vi "Main_Module.vi"(11 "Error_In":errorcluster) -> (15 "Error_Out":errorcluster)   [LabVIEW 2021]
doc: "This is the Main VI for the user to interact with."
uses:
  Controls/Queue_Operation.ctl
  Controls/Logger_Data.ctl
  Controls/Temperature_Limit.ctl
  Controls/Current_Limit.ctl
  Controls/Generated_data.ctl
  Controls/Main_Status.ctl
panel:
  in  "Log_Rate":dbl=1.0 min=1.0 max=120.0
  out "Temperature":dbl
  out "Current":dbl
  out "Generated_Data":dbl[][](graph)
  in  "Exit":bool
  in  "Current_Limit":T1={"Current_High_Limit"=120.0, "Current_Low_Limit"=0.0} caption="Current Limit" {"Current_High_Limit" min=101.0 max=120.0; "Current_Low_Limit" min=100.0 max=119.0}
  in  "Temperature_Limit":T2={"Temperature_High_Limit"=49.0, "Temperature_Low_Limit"=30.0} caption="Temperature Limit" {"Temperature_Low_Limit" min=30.0 max=49.0; "Temperature_High_Limit" min=31.0 max=50.0}
  in  "Start/Stop_Acquisition":bool caption="Start/Stop Acquisition"
  # "ADQ System"
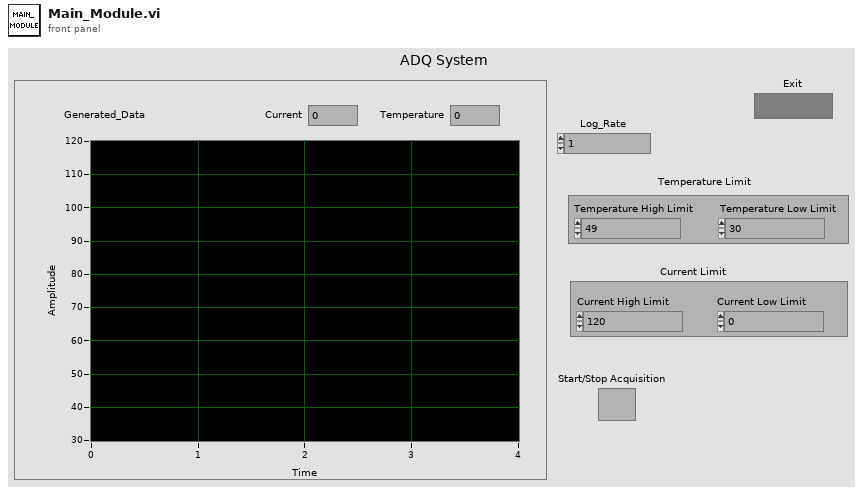
[diagram p1: front panel]
types:
  T1 = typedef "Current_Limit.ctl" = cluster{"Current_High_Limit":dbl, "Current_Low_Limit":dbl}
  T2 = typedef "Temperature_Limit.ctl" = cluster{"Temperature_High_Limit":dbl, "Temperature_Low_Limit":dbl}
  T3 = typedef "Main_Status.ctl" = cluster{"Stop?":bool, "Start/Stop_Acquisition ":bool, "Wait_Time":i32}
  T4 = typedef "Queue_Operation.ctl" = enum16{"Obtain_Queue", "Enqueue", "Lossy_Enqueue", "Preview", "Queue_Status", "Release_Queue", "Dequeue", "Flush"}
  T5 = enum8{"Enabled", "Disabled", "Disabled and Grayed Out"}
  T6 = typedef "Logger_Data.ctl" = cluster{"Generated_Data":T7, "Current_Limit":T1, "Temperature_Limit":T2}
  T7 = typedef "Generated_data.ctl" = cluster{"Current_Data":dbl, "Temp_Data":dbl}
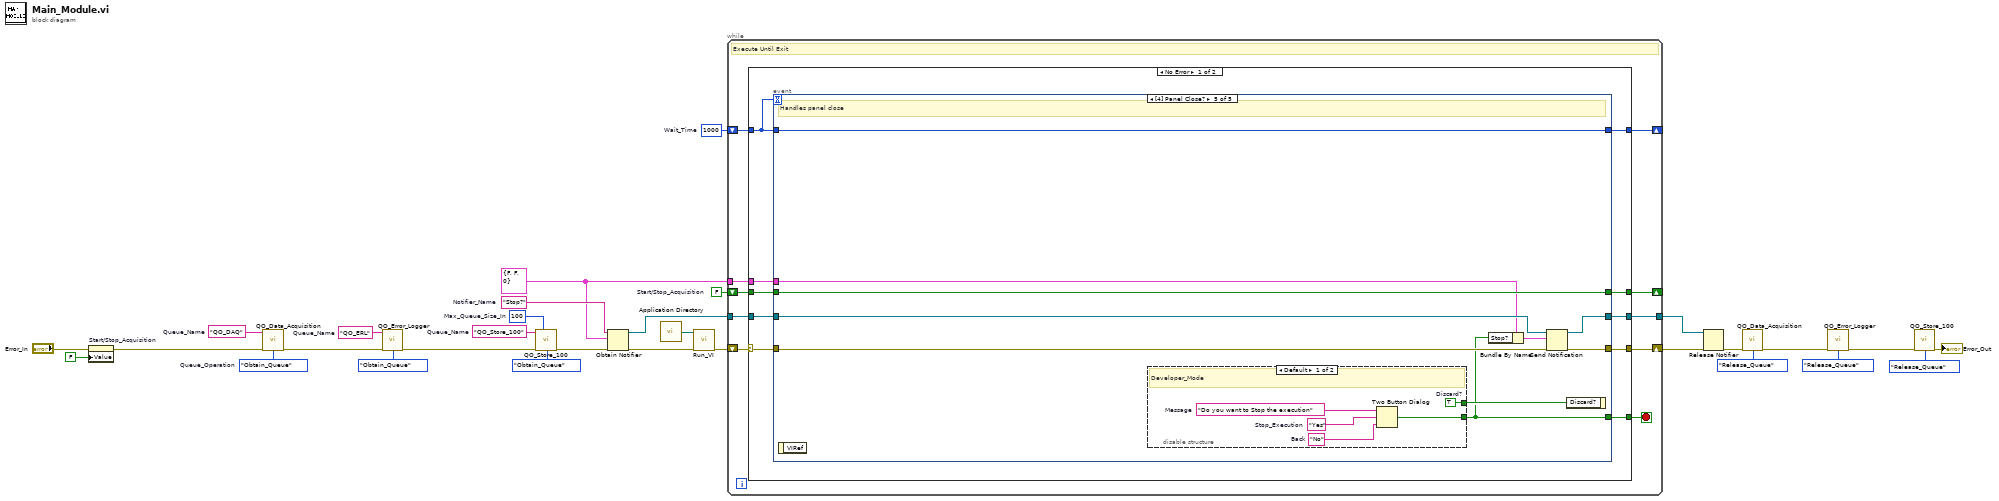
[diagram p0: block diagram]
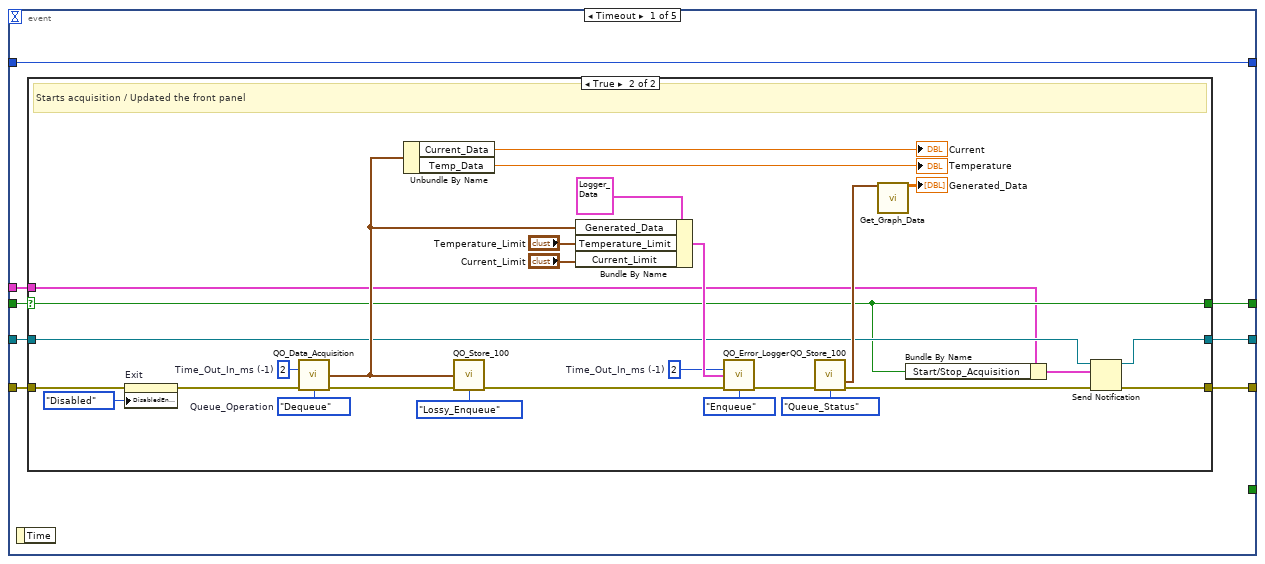
[diagram p2: hidden frame]
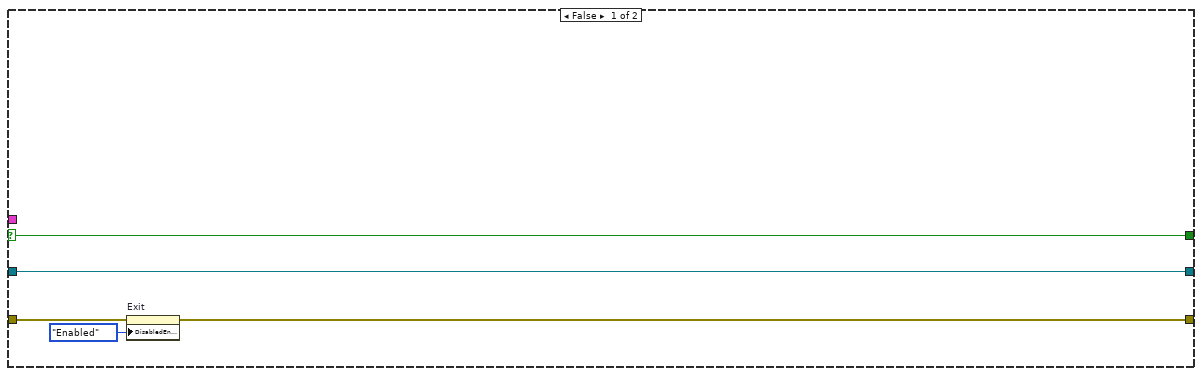
[diagram p3: hidden frame]
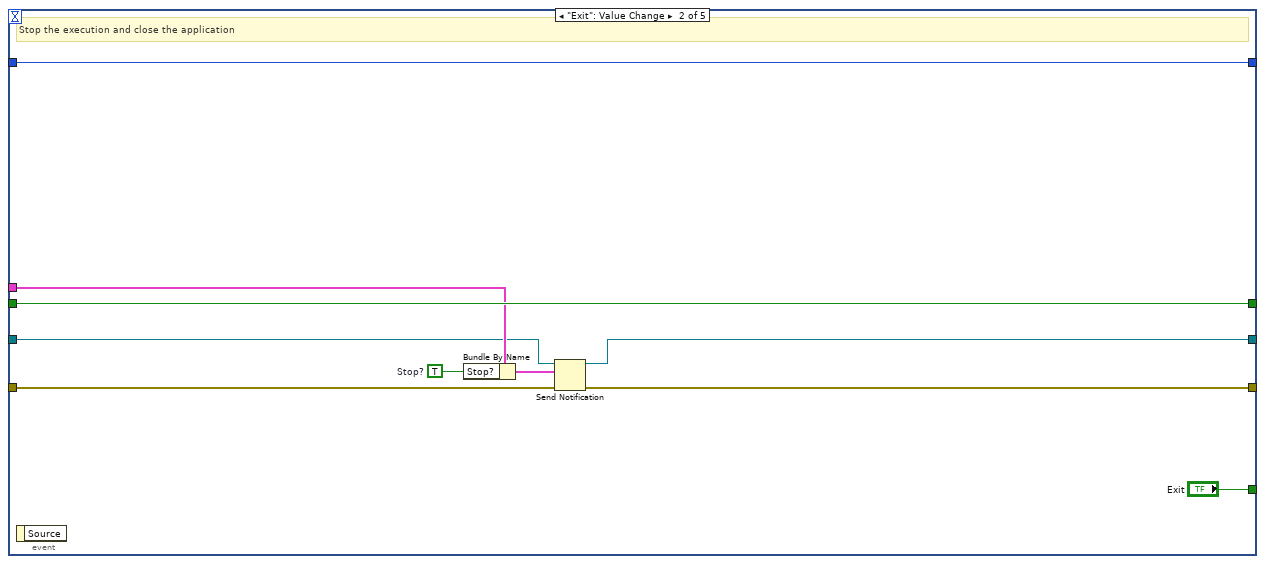
[diagram p4: hidden frame]
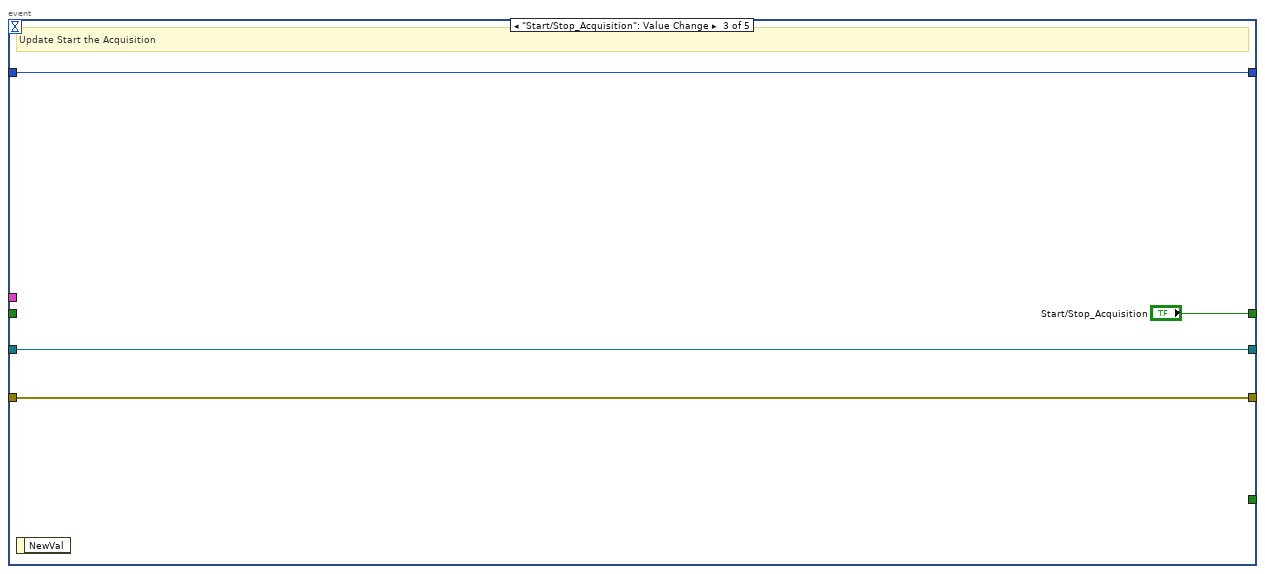
[diagram p5: hidden frame]
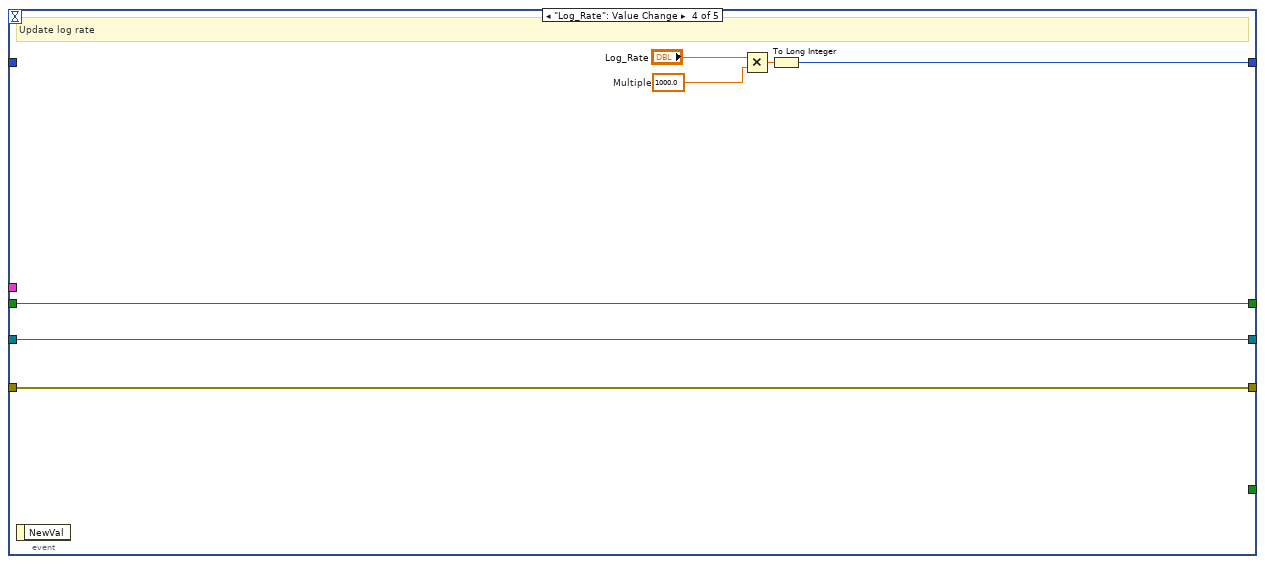
[diagram p6: hidden frame]
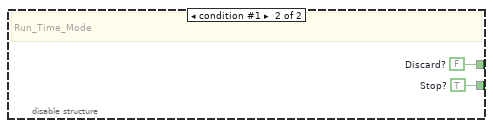
[diagram p7: hidden frame]
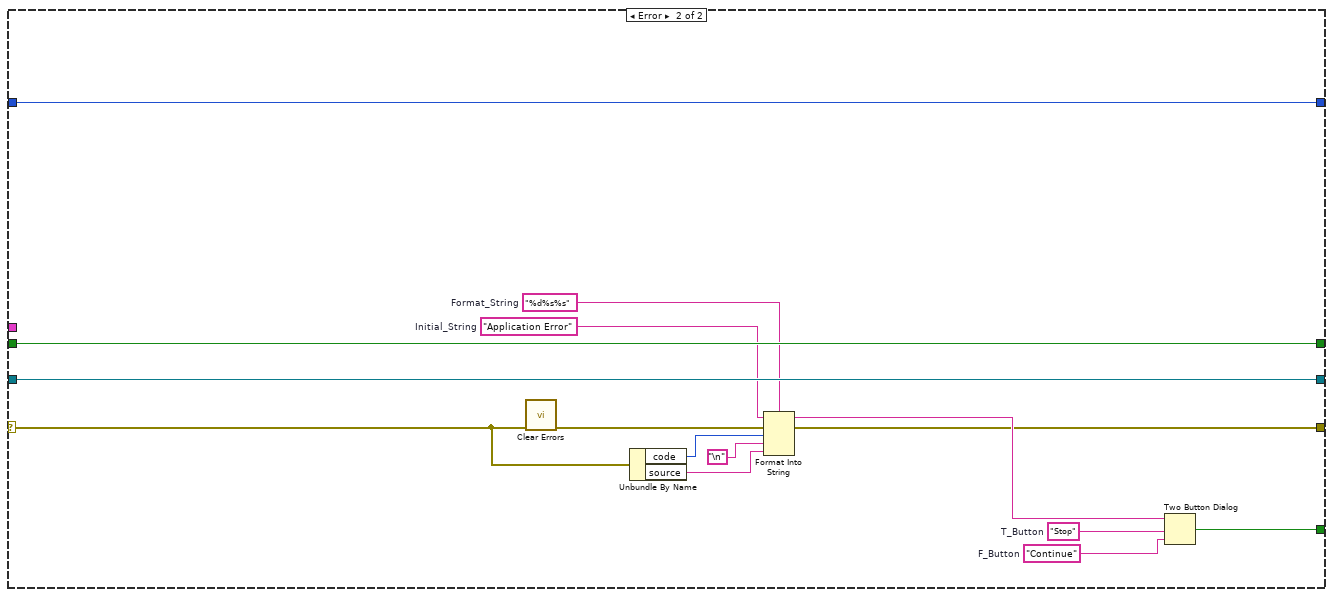
[diagram p8: hidden frame]
diagram:
  w2 = T3 {"Stop?"=FALSE, "Start/Stop_Acquisition "=FALSE, "Wait_Time"=0}
  w11 = "QO_Store_100"  # Queue_Name
  w12 = "QO_ERL"  # Queue_Name
  w13 = "QO_DAQ"  # Queue_Name
  w21 = "Stop?"  # Notifier_Name
  w27 = 1000  # Wait_Time
  w23 = 100  # Max_Queue_Size_In
  w28 = FALSE  # Start/Stop_Acquisition
  w29 = Queue_Operation."Obtain_Queue"  # Queue_Operation
  n1 = property on="Start/Stop_Acquisition" class="Bool (strict)"(error in="Error_In", "Value"=FALSE ("Start/Stop_Acquisition")) -> (error out=w10:errorcluster)  [unwired: 1 in, 1 out]
  n2 = call "QO_Data_Acquisition.vi"("Queue_Name_In"=w13, "Error_In"=w10, "Queue_Operation"=w29) -> ("Error_Out"=w30:errorcluster)  [unwired: 8 in, 4 out]
  n3 = call "QO_Error_Logger.vi"("Queue_Name_In"=w12, "Error_In"=w30, "Queue_Operation"=Queue_Operation."Obtain_Queue") -> ("Error_Out"=w26:errorcluster)  [unwired: 8 in, 4 out]
  n4 = call "QO_Store_100.vi"("Queue_Name_In"=w11, "Max_Queue_Size_In"=w23, "Error_In"=w26, "Queue_Operation"=Queue_Operation."Obtain_Queue") -> ("Error_Out"=w24:errorcluster)  [unwired: 7 in, 4 out]
  n5 = Obtain Notifier(name (unnamed)=w21, notification data type=w2, error in (no error)=w24) -> (notifier out=w20:refnum<notifier>, error out=w17:errorcluster)  [unwired: 1 in, 1 out]
  n6 = call <vilib>:"Application Directory.vi"() -> ("Application Directory"=w15:path)
  n7 = call "Run_VI.vi"("Application_Directory"=w15, "Error_In"=w17) -> ("Error_Out"=w16:errorcluster)  [unwired: 13 in]
  n8 = while {
    shift-right: [w38] -> _
    shift-left: w28 -> [w37]
    shift-right: [w35] -> _
    shift-left: w27 -> [w36]
    tunnel: w20 -> [w34]
    tunnel: [w33] -> w19
    tunnel: w2 -> [w32]
    shift-right: [w31] -> w1
    shift-left: w16 -> [w40]
    stop <- w39 stop-if-true
    # "Execute Until Exit"
    n9 = case shown="No Error" w40 {
      selector: w40 -> [w41 w131]
      tunnel: [w50 w130] -> w39
      tunnel: [w49 w144] -> w38
      tunnel: w37 -> [w48 w144]
      tunnel: [w47 w132] -> w31
      tunnel: w36 -> [w43 w143]
      tunnel: [w46 w143] -> w35
      tunnel: w34 -> [w42 w142]
      tunnel: [w44 w142] -> w33
      tunnel: w32 -> [w45 _]
      frame No Error {
        n10 = event shown="[4] Panel Close?" {
          selector: _ -> [_ _ _ _ _]
          dyn-events: _ -> [_ _ _ _ _]
          timeout: w43 -> [_ _ _ _ _]
          tunnel: [_ "Exit" _ _ w114] -> w50
          tunnel: [w57 w100 "Start/Stop_Acquisition" w106 w121] -> w49
          tunnel: w48 -> [w56 w100 _ w106 w121]
          tunnel: w41 -> [w54 w99 w105 w108 w120]
          tunnel: [w58 w97 w105 w108 w118] -> w47
          tunnel: [w55 w98 w104 w109 w119] -> w46
          tunnel: w43 -> [w55 w98 w104 _ w119]
          tunnel: w45 -> [w51 w94 _ _ w115]
          tunnel: w42 -> [w53 w93 w102 w107 w117]
          tunnel: [w52 w92 w102 w107 w113] -> w44
          event Timeout {
            n11 = event-data() -> ()  [unwired: 1 in, 1 out]
            n12 = case shown="True" w56 {
              selector: w56 -> [w62 w69]
              tunnel: w54 -> [w63 w91]
              tunnel: [w60 w73] -> w58
              tunnel: [w62 w69] -> w57
              tunnel: w53 -> [w61 w72]
              tunnel: [w61 w71] -> w52
              tunnel: w51 -> [_ w68]
              frame False {
                n13 = property on="Exit" class="Bool"(error in=w63, "DisabledEnum"=T5."Enabled" ("Disabled")) -> (error out=w60:errorcluster)  [unwired: 1 in, 1 out]
              }
              frame True {
                w75 = 2  # Time_Out_In_ms (-1)
                w76 = 2  # Time_Out_In_ms (-1)
                w90 = Queue_Operation."Dequeue"  # Queue_Operation
                # "Starts acquisition / Updated the front panel"
                n14 = property on="Exit" class="Bool"(error in=w91, "DisabledEnum"=T5."Disabled" ("Disabled")) -> (error out=w65:errorcluster)  [unwired: 1 in, 1 out]
                n15 = call "QO_Data_Acquisition.vi"("Time_Out_In_ms (-1)"=w76, "Error_In"=w65, "Queue_Operation"=w90) -> ("Data_Out"=w80:T7, "Error_Out"=w88:errorcluster)  [unwired: 8 in, 3 out]
                n16 = Unbundle By Name(w80) -> ("Current_Data"=→"Current":dbl, "Temp_Data"=→"Temperature":dbl)
                n17 = call "QO_Store_100.vi"("Data_In"=w80, "Error_In"=w88, "Queue_Operation"=Queue_Operation."Lossy_Enqueue") -> ("Error_Out"=w77:errorcluster)  [unwired: 8 in, 4 out]
                n18 = Bundle By Name(cluster=T6 {"Generated_Data"={"Current_Data"=0.0, "Temp_Data"=0.0}, "Current_Limit"={"Current_High_Limit"=0.0, "Current_Low_Limit"=0.0}, "Temperature_Limit"={"Temperature_High_Limit"=0.0, "Temperature_Low_Limit"=0.0}} ("Logger_Data"), "Generated_Data"=w80, "Temperature_Limit"="Temperature_Limit", "Current_Limit"="Current_Limit") -> (w82:T6)
                n19 = call "QO_Error_Logger.vi"("Time_Out_In_ms (-1)"=w75, "Data_In"=w82, "Error_In"=w77, "Queue_Operation"=Queue_Operation."Enqueue") -> ("Error_Out"=w84:errorcluster)  [unwired: 7 in, 4 out]
                n20 = call "QO_Store_100.vi"("Error_In"=w84, "Queue_Operation"=Queue_Operation."Queue_Status") -> ("Total_Data"=w85:T7[], "Error_Out"=w74:errorcluster)  [unwired: 9 in, 3 out]
                n21 = call "Get_Graph_Data.vi"("Total_Data"=w85) -> ("Array"=→"Generated_Data":dbl[][])  [unwired: 14 in]
                n22 = Bundle By Name(cluster=w68, "Start/Stop_Acquisition"=w69) -> (w70:T3)
                n23 = Send Notification(notification=w70, notifier=w72, error in (no error)=w74) -> (notifier out=w71:refnum<notifier>, error out=w73:errorcluster)
              }
            }
          }
          event "Exit": Value Change {
            w96 = TRUE  # Stop?
            # "Stop the execution and close the application"
            n24 = event-data() -> ()  [unwired: 1 in, 1 out]
            n25 = Bundle By Name(cluster=w94, "Stop?"=w96) -> (w95:T3)
            n26 = Send Notification(notification=w95, notifier=w93, error in (no error)=w99) -> (notifier out=w92:refnum<notifier>, error out=w97:errorcluster)
          }
          event "Start/Stop_Acquisition": Value Change {
            # "Update Start the Acquisition"
            n27 = event-data() -> ()  [unwired: 1 in, 1 out]
          }
          event "Log_Rate": Value Change {
            w111 = 1000.0  # Multiple
            # "Update log rate"
            n28 = event-data() -> ()  [unwired: 1 in, 1 out]
            n29 = Multiply(x="Log_Rate", y=w111) -> (x*y=w110:dbl)
            n30 = To Long Integer(number=w110) -> (32bit integer=w109:i32)
          }
          event Panel Close? {
            # "Handles panel close"
            n31 = event-data() -> ()  [unwired: 1 in, 1 out]
            n32 = disable-structure shown="Default" {
              disable-tunnel: [w124 w129] -> w114
              disable-tunnel: [w123 w128] -> w122
              frame condition #0 (active) {
                w123 = TRUE  # Discard?
                w125 = "No"  # Back
                w126 = "Yes"  # Stop_Execution
                w127 = "Do you want to Stop the execution"  # Message
                # "Developer_Mode"
                n33 = Two Button Dialog(message=w127, 1:w125, 2:w126) -> (T button?=w124:bool)
              }
              frame condition #1 {
                w128 = FALSE  # Discard?
                w129 = TRUE  # Stop?
                # "Run_Time_Mode"
              }
            }
            n34 = Bundle By Name(cluster=w115, "Stop?"=w114) -> (w116:T3)
            n35 = Send Notification(notification=w116, notifier=w117, error in (no error)=w120) -> (notifier out=w113:refnum<notifier>, error out=w118:errorcluster)
            n36 = event-data("Discard?"=w122) -> ()  [unwired: 1 in, 1 out]
          }
        }
      }
      frame Error {
        w137 = "%d%s%s"  # Format_String
        w138 = "Application Error"  # Initial_String
        w139 = "Stop"  # T_Button
        w140 = "Continue"  # F_Button
        n37 = call <vilib>:"Clear Errors.vi"("error in (no error)"=w131) -> ("error out"=w135:errorcluster)  [unwired: 5 in, 1 out]
        n38 = Unbundle By Name(w131) -> ("code"=w134:i32, "source"=w133:string)
        n39 = Format Into String(format string=w137, initial string=w138, error in=w135, w134, "\n", w133) -> (resulting string=w141:string, error out=w132:errorcluster)
        n40 = Two Button Dialog(message=w141, 1:w140, 2:w139) -> (T button?=w130:bool)
      }
    }
  }
  n41 = Release Notifier(notifier=w19, error in (no error)=w1) -> (error out=w14:errorcluster)  [unwired: 1 in, 2 out]
  n42 = call "QO_Data_Acquisition.vi"("Error_In"=w14, "Queue_Operation"=Queue_Operation."Release_Queue") -> ("Error_Out"=w8:errorcluster)  [unwired: 9 in, 4 out]
  n43 = call "QO_Error_Logger.vi"("Error_In"=w8, "Queue_Operation"=Queue_Operation."Release_Queue") -> ("Error_Out"=w7:errorcluster)  [unwired: 9 in, 4 out]
  n44 = call "QO_Store_100.vi"("Error_In"=w7, "Queue_Operation"=Queue_Operation."Release_Queue") -> ("Error_Out"=→"Error_Out":errorcluster)  [unwired: 9 in, 4 out]
